vi "Initialize-object.vi"(7 "Main VI ref":refnum<vi>, 8 "error in (no error)":errorcluster) -> (0 "error out":errorcluster, 3 "Object ref out":T1)   [LabVIEW 2013, in "HardwareCharacterization.lvlib" / "HC-Main.lvclass"]
uses:
  HC-Main.lvclass
  Object-reference.ctl
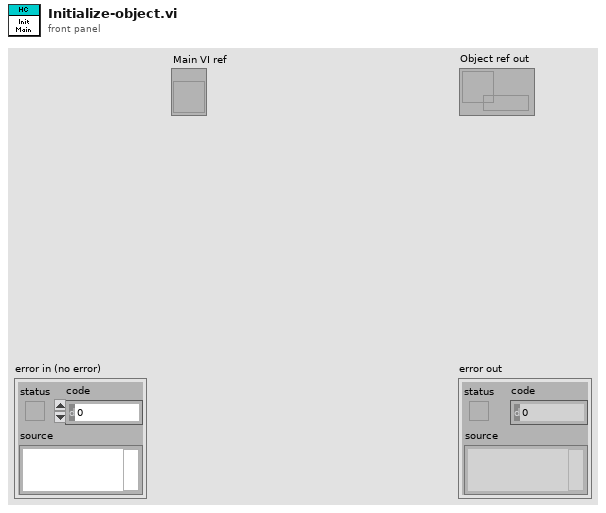
[diagram p1: front panel]
types:
  T1 = typedef "HardwareCharacterization.lvlib/HC-Main.lvclass/Object-reference.ctl" = refnum<data-value>
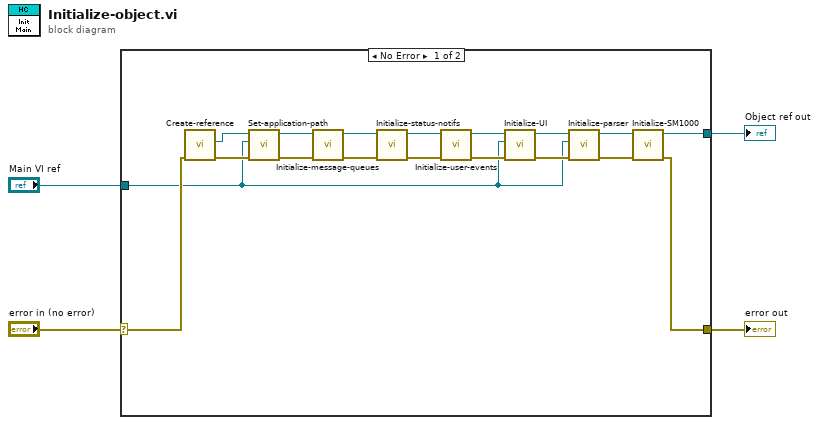
[diagram p0: block diagram]
diagram:
  n1 = case shown="No Error" "error in (no error)" {
    selector: "error in (no error)" -> [w16 w23]
    tunnel: [w11 w23] -> w3
    tunnel: [w10 _] -> w2
    tunnel: "Main VI ref" -> [w5 _]
    frame No Error {
      n2 = call "Create-reference.vi"("error in (no error)"=w16) -> ("error out"=w15:errorcluster, "Data ref"=w12:T1)  [unwired: 8 in, 1 out]
      n3 = call "Set-application-path.vi"("error in (no error)"=w15, "Main VI ref"=w5, "Data ref. in"=w12) -> ("error out"=w13:errorcluster, "Data ref."=w14:T1)  [unwired: 7 in]
      n4 = call "Initialize-message-queues.vi"("error in (no error)"=w13, "Object ref in"=w14) -> ("error out"=w19:errorcluster, "Object ref out"=w22:T1)  [unwired: 8 in]
      n5 = call "Initialize-status-notifs.vi"("error in (no error)"=w19, "Object ref in"=w22) -> ("error out"=w18:errorcluster, "Object ref out"=w21:T1)  [unwired: 8 in]
      n6 = call "Initialize-user-events.vi"("error in (no error)"=w18, "Object ref in"=w21) -> ("error out"=w17:errorcluster, "Object ref out"=w20:T1)  [unwired: 8 in]
      n7 = call "Initialize-UI.vi"("error in (no error)"=w17, "Main VI ref"=w5, "Object ref in"=w20) -> ("error out"=w7:errorcluster, "Object ref out"=w8:T1)  [unwired: 7 in]
      n8 = call "Initialize-parser.vi"("error in (no error)"=w7, "Main VI ref"=w5, "Data ref. in"=w8) -> ("error out"=w6:errorcluster, "Data ref."=w9:T1)  [unwired: 7 in]
      n9 = call "Initialize-SM1000.vi"("error in (no error)"=w6, "Data ref. in"=w9) -> ("error out"=w11:errorcluster, "Data ref."=w10:T1)  [unwired: 8 in]
    }
    frame Error {
    }
  }
  "error out" <- w3
  "Object ref out" <- w2
